vi "Oxford Command With Checking.vi"(3 "error in (no error)":errorcluster, 4 "Command":string="@0V", 5 "VISA session":refnum<visa-resource-name>) -> (0 "error out":errorcluster, 1 "String Read":string, 2 "dup VISA session":refnum<visa-resource-name>)   [LabVIEW 2019]
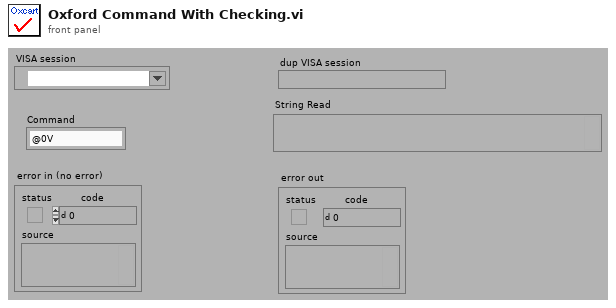
[diagram p1: front panel]
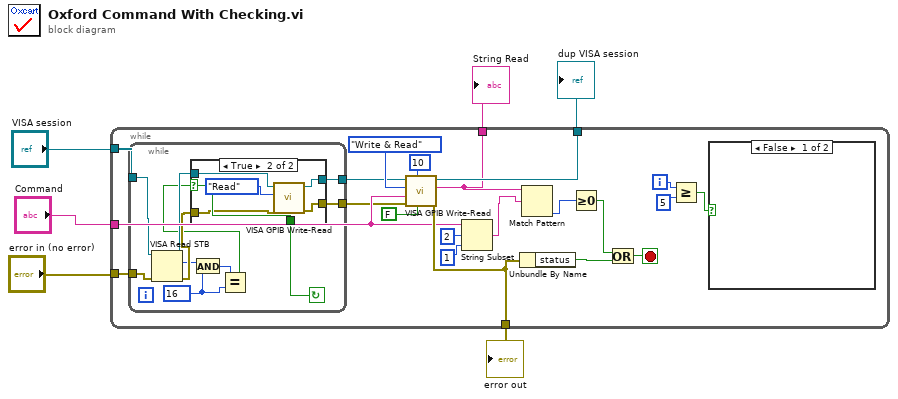
[diagram p0: block diagram]
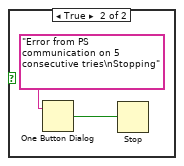
[diagram p3: hidden frame]
diagram:
  n1 = while {
    tunnel: "Command" -> [w22]
    tunnel: "error in (no error)" -> [w10]
    tunnel: [w26] -> w4
    tunnel: [w23] -> w3
    tunnel: "VISA session" -> [w11]
    tunnel: [w14] -> w1
    i -> [w18]
    stop <- w19 stop-if-true
    n2 = while {
      tunnel: w11 -> [w38]
      tunnel: w10 -> [w34]
      tunnel: [w36] -> w9
      tunnel: [w35] -> w8
      stop <- w30 continue-if-true
      w29 = u16 16 ("y")
      n3 = VISA Read STB(8:w34, 11:w38) -> (0:w33:errorcluster, 2:w32:u16, 3:w37:refnum<visa-resource-name>)
      n4 = And(x=w32, y=w29) -> (x .and. y?=w31:u16)
      n5 = Equal?(x=w31, y=w29) -> (x = y?=w28:bool)
      n6 = case shown="True" w28 {
        selector: w28 -> [w41 w45]
        tunnel: w37 -> [w40 w46]
        tunnel: [w41 w45] -> w30
        tunnel: [w39 w44] -> w36
        tunnel: [w40 w43] -> w35
        tunnel: w33 -> [w39 w42]
        frame False {
        }
        frame True {
          n7 = call "VISA GPIB Write-Read.vi"("error in (no error)"=w42, "Action"=enum16{"Write", "Read", "Write & Read"}."Read", "VISA resource name"=w46) -> ("error out"=w44:errorcluster, "dup VISA Session"=w43:refnum<visa-resource-name>)  [unwired: 5 in, 2 out]
        }
      }
    }
    n8 = call "VISA GPIB Write-Read.vi"("Wait For SRQ"=FALSE, "Wait (ms)"=u32 10 ("wait (mS)"), "error in (no error)"=w9, "Command"=w22, "Action"=enum16{"Write", "Read", "Write & Read"}."Write & Read", "VISA resource name"=w8) -> ("error out"=w26:errorcluster, "String Returned"=w14:string, "dup VISA Session"=w23:refnum<visa-resource-name>)  [unwired: 2 in, 1 out]
    n9 = String Subset(string=w22, offset (0)=2, length (rest)=1 ("length (rest)")) -> (substring=w13:string)
    n10 = Unbundle By Name(w26) -> ("status"=w24:bool)
    n11 = Match Pattern(string=w14, regular expression=w13) -> (offset past match=w12:i32)  [unwired: 1 in, 3 out]
    n12 = Greater Or Equal To 0?(x=w12) -> (x >= 0?=w25:bool)
    n13 = Or(x=w25, y=w24) -> (x .or. y?=w19:bool)
    n14 = Greater Or Equal?(x=w18, y=5) -> (x >= y?=w16:bool)
    n15 = case shown="False" w16 {
      frame False {
      }
      frame True {
        n16 = One Button Dialog(message="Error from PS communication on 5 consecutive tries\nStopping") -> (true=w48:bool)  [unwired: 1 in]
        n17 = Stop(stop? (T)=w48) -> ()
      }
    }
  }
  "error out" <- w4
  "String Read" <- w1
  "dup VISA session" <- w3
